vi "Multichannel Read Example.vi"() -> ()   [LabVIEW 2014]
uses:
  <vilib>/_DAQmxBase/Internals/DAQmxBase Create Channel (AI-Voltage-Basic).vi
  <vilib>/_DAQmxBase/Internals/DAQmxBase Read (Analog 2D DBL NChan NSamp).vi
panel:
  in  "stop":bool
  out "Waveform Graph":dbl[][](graph)
  in  "physical channels":tag
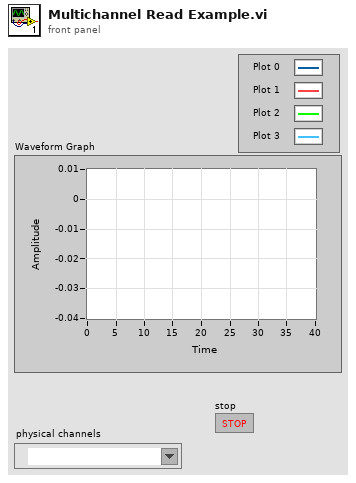
[diagram p1: front panel]
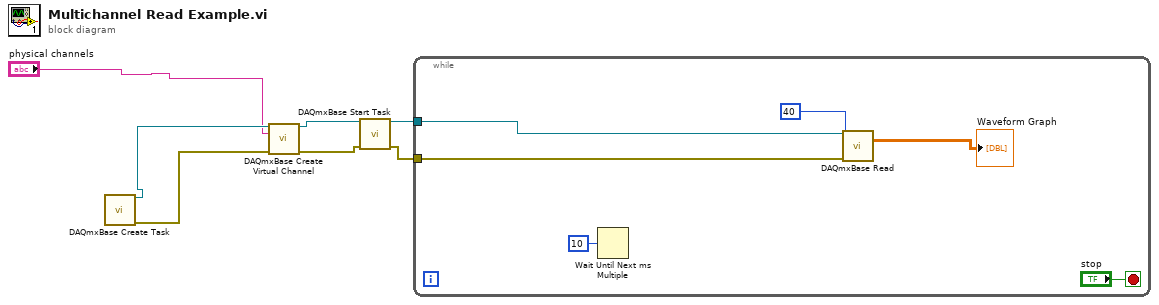
[diagram p0: block diagram]
diagram:
  n1 = call <vilib>:"DAQmxBase Create Task.vi"() -> ("task out"=w3:refnum<k21>, "error out"=w2:errorcluster)  [unwired: 14 in]
  n2 = call-poly <vilib>:"DAQmxBase Create Virtual Channel.vi"("task in"=w3, "physical channels"="physical channels", "error in"=w2) -> ("task out"=w6:refnum<k21>, "error out"=w7:errorcluster)  [unwired: 11 in]
  n3 = call <vilib>:"DAQmxBase Start Task.vi"("task/channels in"=w6, "error in"=w7) -> ("task out"=w5:refnum<k21>, "error out"=w4:errorcluster)  [unwired: 12 in]
  n4 = while {
    tunnel: w5 -> [w10]
    tunnel: w4 -> [w9]
    stop <- "stop" stop-if-true
    n5 = Wait Until Next ms Multiple(millisecond multiple=u32 10) -> ()  [unwired: 1 out]
    n6 = call-poly <vilib>:"DAQmxBase Read.vi"("task/channels in"=w10, "number of samples per channel"=40, "error in"=w9) -> ("data"=→"Waveform Graph":dbl[][])  [unwired: 10 in, 2 out]
  }
